vi "Reach_Current_Target.vi"(8 "error in (no error)":errorcluster, 10 "Amps":dbl, 11 "VISA Refnum in":refnum<visa-resource-name>) -> (0 "error out":errorcluster, 2 "Laser current":dbl caption="Current", 3 "VISA Refnum out":refnum<visa-resource-name>)   [LabVIEW 2024]
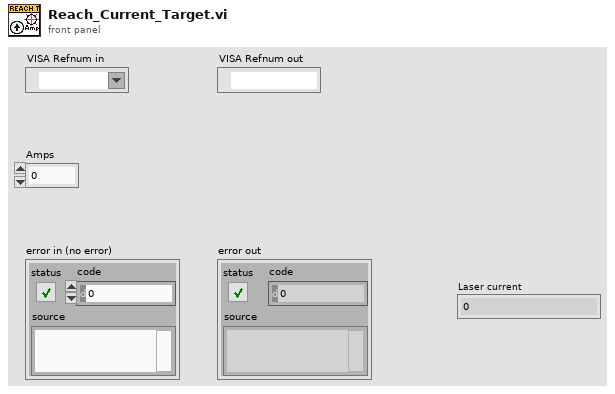
[diagram p1: front panel]
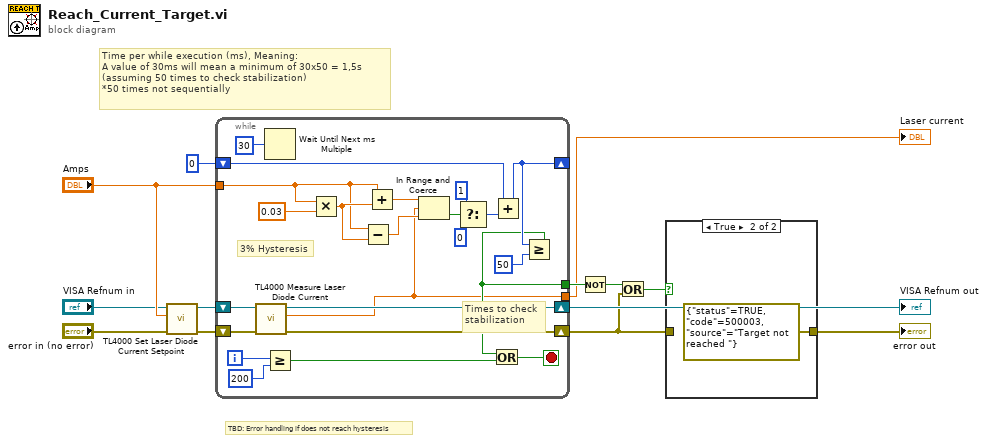
[diagram p0: block diagram]
diagram:
  # "Time per while execution (ms), Meaning:\nA value of 30ms will mean a minimum of 30x50 = 1,5s \n(assuming 50 times to check stabilization)\n*50 times not sequentially"
  # "TBD: Error handling if does not reach hysteresis"
  n1 = call <instrlib>:"TL4000 Set Laser Diode Current Setpoint.vi"("error in (no error)"="error in (no error)", "Laser Diode Current Setpoint (0.0)"="Amps", "instrument handle"="VISA Refnum in") -> ("error out"=w10:errorcluster, "instrument handle out"=w9:refnum<visa-resource-name>)  [unwired: 7 in]
  n2 = while {
    shift-right: [w33] -> w11
    shift-left: w9 -> [w36]
    shift-right: [w34] -> w4
    shift-left: w10 -> [w35]
    tunnel: "Amps" -> [w28]
    shift-right: [w21] -> _
    shift-left: 0 -> [w24]
    tunnel: [w15] -> w5
    tunnel: [w14] -> w1
    i -> [w19]
    stop <- w16 stop-if-true
    # "Times to check\nstabilization"
    # "3% Hysteresis"
    n3 = call <instrlib>:"TL4000 Measure Laser Diode Current.vi"("error in (no error)"=w35, "instrument handle"=w36) -> ("error out"=w34:errorcluster, "Current"=w14:dbl, "instrument handle out"=w33:refnum<visa-resource-name>)  [unwired: 7 in]
    n4 = Wait Until Next ms Multiple(millisecond multiple=u32 30 ("milliseconds to wait")) -> ()  [unwired: 1 out]
    n5 = Greater Or Equal?(x=w19, y=200) -> (x >= y?=w17:bool)
    n6 = Multiply(x=w28, y=0.03) -> (x*y=w30:dbl)
    n7 = Subtract(x=w28, y=w30) -> (x-y=w29:dbl)
    n8 = Add(x=w28, y=w30) -> (x+y=w31:dbl)
    n9 = In Range and Coerce(upper limit=w31, x=w14, lower limit=w29) -> (In Range?=w27:bool)  [unwired: 1 out]
    n10 = Select(t=1, s=w27, f=0) -> (s? t:f=w25:i32)
    n11 = Add(x=w24, y=w25) -> (x+y=w21:i32)
    n12 = Greater Or Equal?(x=w21, y=50) -> (x >= y?=w15:bool)
    n13 = Or(x=w15, y=w17) -> (x .or. y?=w16:bool)
  }
  "VISA Refnum out" <- w11
  "Laser current" <- w1
  n14 = Not(x=w5) -> (.not. x?=w3:bool)
  n15 = Or(x=w3, y=w4) -> (x .or. y?=w2:bool)
  n16 = case shown="True" w2 {
    tunnel: w4 -> [w37 _]
    tunnel: [w37 errorcluster {"status"=TRUE, "code"=500003, "source"="Target not reached "} ("error constant")] -> w6
    frame False {
    }
    frame True {
    }
  }
  "error out" <- w6
